vi "子VI-读取缺陷测量长宽和面积.vi"(10 "Particle Reports (Pixels)":T1(array[cluster]) {"Orientation" format="%.2f"; "Dimensions"."Height" format="%.2f"; "Dimensions"."Width" format="%.2f"; "Center of Mass"."Y" format="%.2f"; "Center of Mass"."X" format="%.2f"; "Bounding Rect"."Bottom" format="%.2f"; "Bounding Rect"."Right" format="%.2f"; "Bounding Rect"."Top" format="%.2f"; "Bounding Rect"."Left" format="%.2f"; "Number of Holes" format="%.2f"; "Area" format="%.2f"}) -> (2 "测量结果":dbl[][](array[numeric]))   [LabVIEW 2018]
panel:
  out "补五列空数字":dbl[](array[numeric])
  out "高":dbl[](array[numeric])
  out "宽":dbl[](array[numeric])
  out "面积":dbl[](array[numeric])
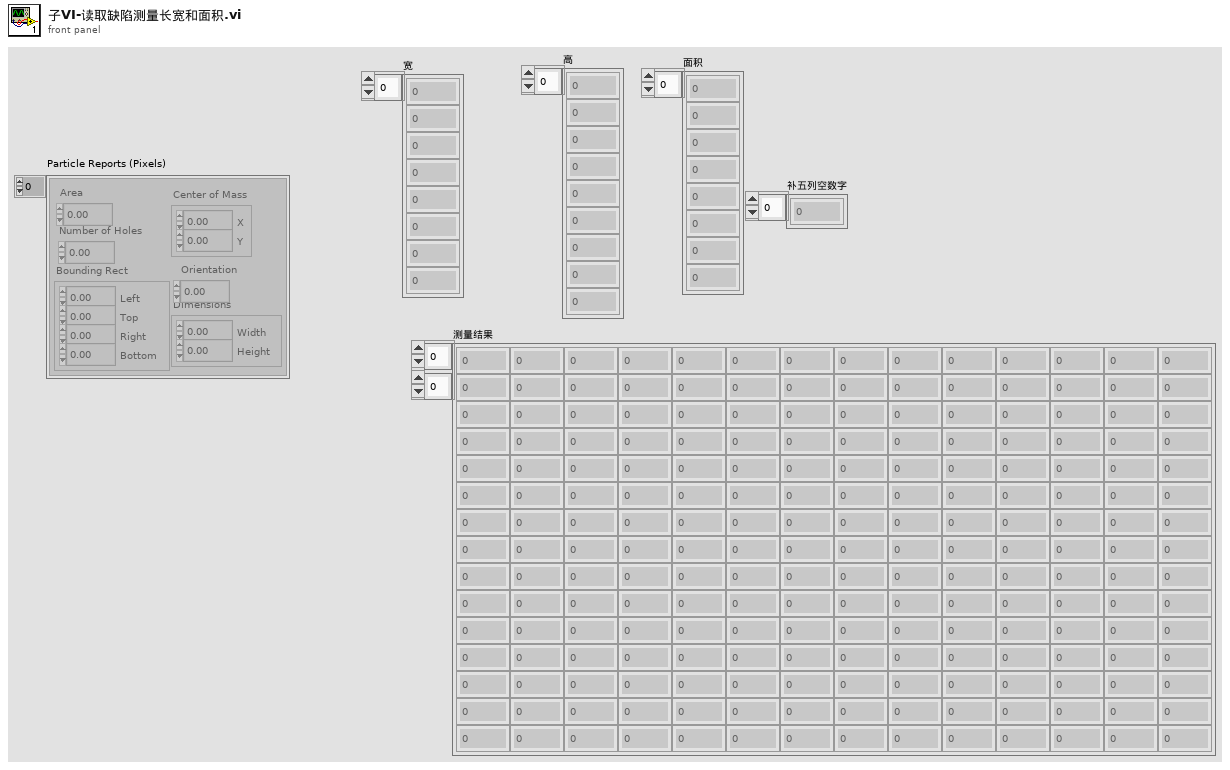
[diagram p1: front panel]
types:
  T1 = cluster{"Area":dbl, "Number of Holes":dbl, "Bounding Rect":cluster{"Left":dbl, "Top":dbl, "Right":dbl, "Bottom":dbl}, "Center of Mass":cluster{"X":dbl, "Y":dbl}, "Orientation":dbl, "Dimensions":cluster{"Width":dbl, "Height":dbl}}[]
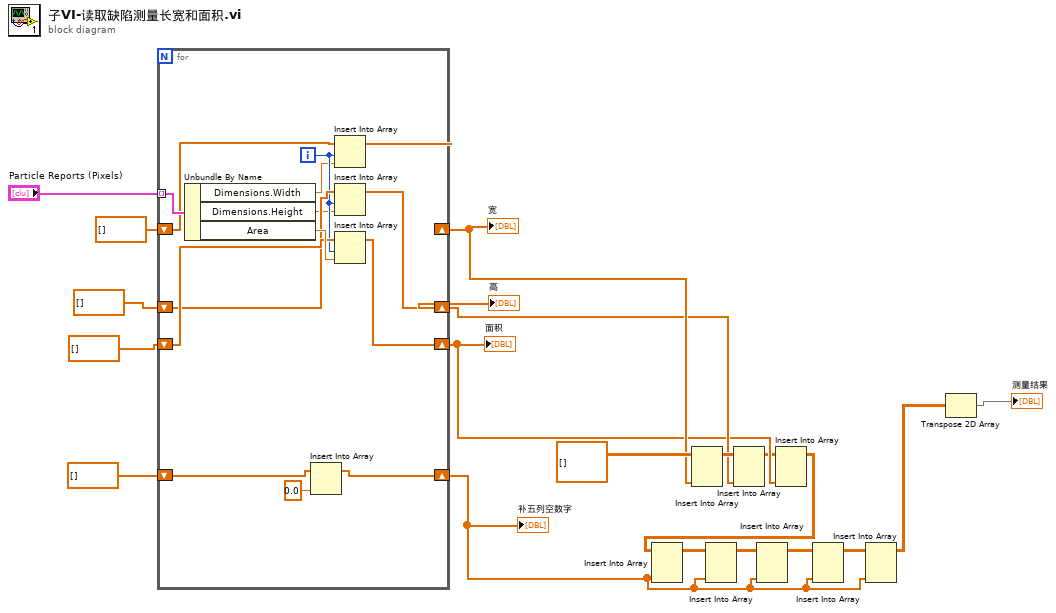
[diagram p0: block diagram]
diagram:
  n1 = for {
    tunnel: "Particle Reports (Pixels)" -> [w33] mode=indexing
    shift-right: [w30] -> w11
    shift-left: dbl[] [] ("数组") -> [w31]
    shift-right: [w25] -> w14
    shift-left: dbl[] [] ("数组") -> [w27]
    shift-right: [w26] -> w12
    shift-left: dbl[] [] ("数组") -> [w29]
    shift-right: [w20] -> w1
    shift-left: dbl[] [] ("数组") -> [w22]
    i -> [w28]
    n2 = Unbundle By Name(w33) -> ("Dimensions.Width"=w23:dbl, "Dimensions.Height"=w24:dbl, "Area"=w32:dbl)
    n3 = Insert Into Array(array=w22, new element=0.0 ("新元素/子数组")) -> (w20:dbl[])  [unwired: 1 in]
    n4 = Insert Into Array(array=w27, index=w28, new element=w23) -> (w25:dbl[])
    n5 = Insert Into Array(array=w29, index=w28, new element=w24) -> (w26:dbl[])
    n6 = Insert Into Array(array=w31, index=w28, new element=w32) -> (w30:dbl[])
  }
  "面积" <- w11
  "宽" <- w14
  "高" <- w12
  "补五列空数字" <- w1
  n7 = Insert Into Array(array=dbl[][] [] ("数组"), new element=w14) -> (w13:dbl[][])  [unwired: 2 in]
  n8 = Insert Into Array(array=w13, new element=w12) -> (w10:dbl[][])  [unwired: 2 in]
  n9 = Insert Into Array(array=w10, new element=w11) -> (w7:dbl[][])  [unwired: 2 in]
  n10 = Insert Into Array(array=w7, new element=w1) -> (w6:dbl[][])  [unwired: 2 in]
  n11 = Insert Into Array(array=w6, new element=w1) -> (w5:dbl[][])  [unwired: 2 in]
  n12 = Insert Into Array(array=w5, new element=w1) -> (w4:dbl[][])  [unwired: 2 in]
  n13 = Insert Into Array(array=w4, new element=w1) -> (w3:dbl[][])  [unwired: 2 in]
  n14 = Insert Into Array(array=w3, new element=w1) -> (w2:dbl[][])  [unwired: 2 in]
  n15 = Transpose 2D Array(2D array=w2) -> (transposed array=→"测量结果":dbl[][])
